vi "Retriggerable Pulse Train.vi"() -> ()   [LabVIEW 2009]
uses:
  <vilib>/DAQmx/configure/trigger.llb/DAQmx Start Trigger (Digital Edge).vi
  <vilib>/DAQmx/configure/timing.llb/DAQmx Timing (Implicit).vi
  <vilib>/DAQmx/create/channels.llb/DAQmx Create Channel (CO-Pulse Generation-Frequency).vi
  Program Files/National Instruments/LabVIEW 2009/resource/objmgr/daqmx.rc
panel:
  in  "samples per channel":i32=5
  in  "stop":bool
  in  "initial delay":dbl format="%.6f"
  in  "idle state":i32(ring)=10214 items=["High"=10192, "Low"=10214]
  in  "counter":tag
  in  "frequency":dbl=1.0 format="%.6f"
  in  "duty cycle":dbl=0.5 format="%.6f"
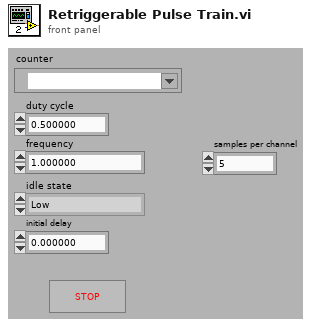
[diagram p1: front panel]
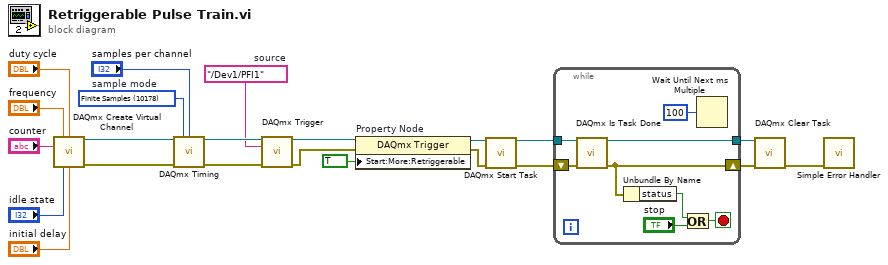
[diagram p0: block diagram]
diagram:
  w6 = tag "/Dev1/PFI1"  # source
  w10 = 10178 items=["Finite Samples"=10178, "Continuous Samples"=10123]  # sample mode
  n1 = call-poly <vilib>:"DAQmx Create Virtual Channel.vi"("frequency"="frequency", "duty cycle"="duty cycle", "counter"="counter", "idle state"="idle state", "initial delay"="initial delay") -> ("task out"=w12:refnum<k21>, "error out"=w11:errorcluster)  [unwired: 9 in]
  n2 = call-poly <vilib>:"DAQmx Timing.vi"("task/channels in"=w12, "sample mode"=w10, "samples per channel"="samples per channel", "error in"=w11) -> ("task out"=w8:refnum<k21>, "error out"=w7:errorcluster)  [unwired: 10 in]
  n3 = call-poly <vilib>:"DAQmx Trigger.vi"("task/channels in"=w8, "source"=w6, "error in"=w7) -> ("task out"=w5:refnum<k21>, "error out"=w4:errorcluster)  [unwired: 11 in]
  n4 = property on="Property Node" class="DAQmx Trigger"(reference=w5, error in=w4, "Start:More:Retriggerable"=TRUE ("Start.Retriggerable")) -> (reference out=w2:refnum<k21>, error out=w1:errorcluster)
  n5 = call <vilib>:"DAQmx Start Task.vi"("task/channels in"=w2, "error in"=w1) -> ("task out"=w17:refnum<k21>, "error out"=w16:errorcluster)  [unwired: 12 in]
  n6 = while {
    tunnel: w17 -> [w30]
    tunnel: [w28] -> w15
    shift-right: [w27] -> w14
    shift-left: w16 -> [w29]
    stop <- w24 stop-if-true
    n7 = call <vilib>:"DAQmx Is Task Done.vi"("task/channels in"=w30, "error in"=w29) -> ("task out"=w28:refnum<k21>, "error out"=w27:errorcluster)  [unwired: 11 in, 1 out]
    n8 = Unbundle By Name "Unbundle By Name"(w27) -> ("status"=w26:bool)
    n9 = Or(x=w26, y="stop") -> (x .or. y?=w24:bool)
    n10 = Wait Until Next ms Multiple(millisecond multiple=u32 100) -> ()  [unwired: 1 out]
  }
  n11 = call <vilib>:"DAQmx Clear Task.vi"("task in"=w15, "error in"=w14) -> ("error out"=w13:errorcluster)  [unwired: 13 in]
  n12 = call <vilib>:"Simple Error Handler.vi"("error in (no error)"=w13) -> ()  [unwired: 4 in, 5 out]
